vi "ReadNet_Darknet.vi"(8 "error in":errorcluster, 10 "DarknetModel":path, 11 "CfgFile":path) -> (0 "error out":errorcluster, 3 "NET":refnum<class "NET.lvclass">)   [LabVIEW 2020, in "OpenLvVision_OpenCv.lvlib"]
doc: "Reads a network model stored in Darknet model files."
uses:
  OpenLvVision_OpenCv.lvlib
  NET/NET.lvclass
  _LvHelpers/EdvrObject/TypeDef/Edvr.ctl
  _LvHelpers/EdvrObject/EdvrObject.lvclass
  Dlls/OlvOpenCvWrapper.dll
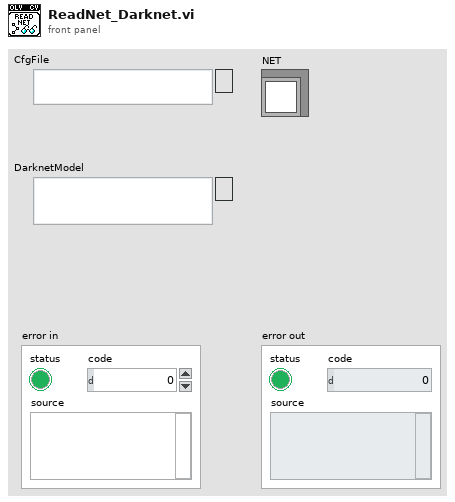
[diagram p1: front panel]
types:
  T1 = typedef "OpenLvVision_OpenCv.lvlib/EdvrObject.lvclass/Edvr.ctl" = refnum<data-value>
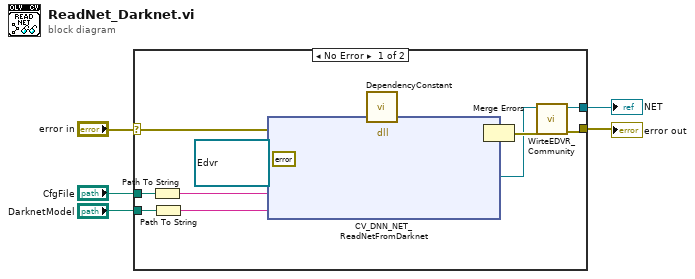
[diagram p0: block diagram]
diagram:
  n1 = case shown="No Error" "error in" {
    selector: "error in" -> [w14 w19]
    tunnel: [w12 w19] -> w4
    tunnel: [w10 _] -> w3
    tunnel: "CfgFile" -> [w9 _]
    tunnel: "DarknetModel" -> [w7 _]
    frame No Error {
      n2 = Path To String(path=w9) -> (string=w8:string)
      n3 = Path To String(path=w7) -> (string=w6:string)
      n4 = dll-call lib="C:/Users/lukas/Downloads/OpenLvVision_OpenCv/SourceCode/LabView/OpenLvVision_OpenCv/Dlls/OlvOpenCvWrapper.dll" fn="CV_DNN_NET_ReadNetFromDarknet"(error in=w14, "Error"=errorcluster {"status"=FALSE, "code"=0, "source"=""} ("error out"), "edvrRef"=T1 refnum ("Edvr"), "cfgFile"=w8, "darknetModel"=w6) -> (error out=w17:errorcluster, "Error"=w16:errorcluster, "edvrRef"=w11:T1)  [unwired: 5 in, 1 out]
      n5 = call "DependencyConstant.vi"() -> ()  [unwired: 12 in]
      n6 = Merge Errors(w17, w16) -> (w13:errorcluster)
      n7 = call "WirteEDVR_Community.vi"("error in"=w13, "Edvr"=w11) -> ("error out"=w12:errorcluster, "NET"=w10:refnum<class "NET.lvclass">)  [unwired: 8 in]
    }
    frame Error {
    }
  }
  "NET" <- w3
  "error out" <- w4
